vi "ConditionalBoolean.vi"(1 "Bool In":bool) -> (0 "Stop?":bool)   [LabVIEW 2020]
doc: "Displays the value of the Boolean indicator and allows conditional breakpoints."
panel:
  in  "Tab Control":enum32{"Data ", "Condition    "}(tab)
  out "Boolean Indicator":bool
  in  "false":bool
  in  "True":bool
  # "Pause If:"
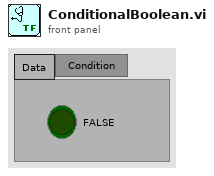
[diagram p1: front panel]
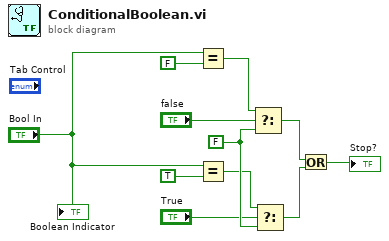
[diagram p0: block diagram]
diagram:
  w10 = FALSE ("f")
  n1 = Equal?(x="Bool In", y=FALSE ("f")) -> (x = y?=w3:bool)
  n2 = Equal?(x="Bool In", y=TRUE ("f")) -> (x = y?=w8:bool)
  n3 = Select(t=w3, s="false", f=w10) -> (s? t:f=w7:bool)
  n4 = Select(t=w8, s="True", f=w10) -> (s? t:f=w6:bool)
  n5 = Or(x=w7, y=w6) -> (x .or. y?=→"Stop?":bool)
  "Boolean Indicator" <- "Bool In"
